vi "test_mass_damper.vi"() -> ()   [LabVIEW 2014]
uses:
  <vilib>/ptbypt/NI_PtbyPt.lvlib
panel:
  in  "B":dbl=10.0 format="%#_13g"
  in  "Mass":dbl=1.0 format="%#_13g"
  in  "Reset":bool
  in  "f(t)":dbl
  in  "stop":bool
  out "reference vs actual":dbl(graph)
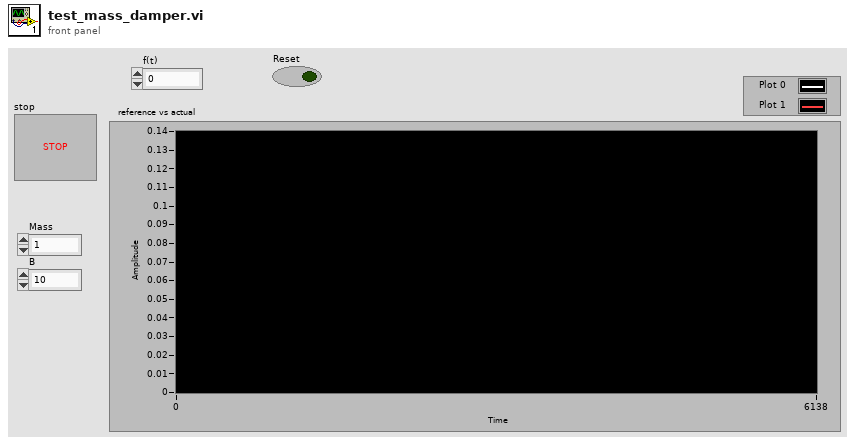
[diagram p1: front panel]
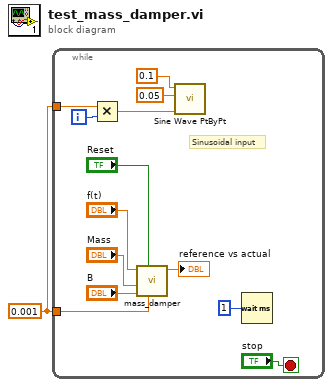
[diagram p0: block diagram]
diagram:
  w1 = 0.001 ("T")
  n1 = while {
    tunnel: w1 -> [w9]
    tunnel: w1 -> [w3]
    i -> [w10]
    stop <- "stop" stop-if-true
    # "Sinusoidal input"
    n2 = Multiply(x=w9, y=w10) -> (x*y=w13:dbl)
    n3 = call "mass_damper.vi"("dt"=w3, "Reset"="Reset", "B"="B", "Mass"="Mass", "f(t)"="f(t)") -> ("x(t)"=→"reference vs actual":dbl)  [unwired: 4 in, 2 out]
    n4 = call <vilib>:"Sine Wave PtByPt.vi"("time"=w13, "frequency"=0.05, "amplitude"=0.1) -> ()  [unwired: 1 in, 1 out]
    n5 = Wait (ms)(milliseconds to wait=u32 1) -> ()  [unwired: 1 out]
  }
